vi "Set Lo Press.vi"(5 "Data.Direction":T1, 6 "leak":bool, 7 "init":bool, 8 "error in (no error)":errorcluster, 11 "Stand in":refnum<class "Stand.lvclass">) -> (0 "error out":errorcluster, 2 "Done":bool)   [LabVIEW 2019, in "Stand.lvclass"]
uses:
  Stand.lvclass
  C:/Users/ANENKOV_V1/Desktop/src/Device_class/Device.lvclass
  TypeDef/Direction.ctl
  Valve DIR.ctl
  Device_class/Device.lvclass/Device.ctl
  1305f1be-f95d-4b4d-845f-89e56356c3b4.vi
  Device_class/GetFPGA.vi
  DoValve.vi
  DoValve.vi/e7d2c9dc-ba67-4685-b926-bcce34aa2778.vi
  DoValve.vi/628819af-fd07-4303-9780-3ddd467101db.vi
  Const All Valve.vi
  FPGA_API_class/FPGA API.lvclass
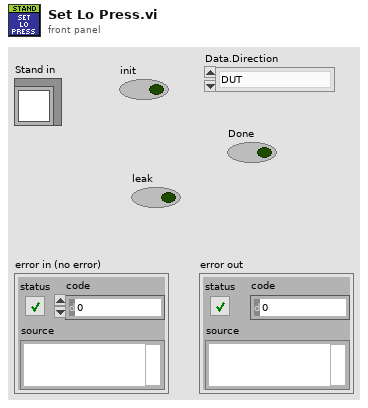
[diagram p1: front panel]
types:
  T1 = typedef "Direction.ctl" = enum8{"DUT", "Chamber"}
  T2 = typedef "Valve DIR.ctl" = enum16{"Air Valves: Open (DUT Filling)", "Air Valves: Open (Chamber Filling)", "Air Valves: Open (Pump Pressure DUT)", "Air Valves: Open (Pump Pressure Chamber)", "Air Valves: Open (Haskel Pressure DUT)", "Air Valves: Open (Haskel Pressure Chamber)", "Air Valves: Open (Slow Release DUT)", "Air Valves: Open (Slow Release Chamber)", "Air Valves: Open (Fast Release DUT)", "Air Valves: Open (Fast Release Chamber)", "Air Valves: Open (Emergency Release DUT and Chamber)", "Air Valves: Leak Hi (Chamber)", "Air Valves: Leak Hi (DUT)", "Air Valves: Backpressure (Chamber)", "Air Valves: Backpressure (DUT)", "Air Valves: Fully Closed", "Air Valves: Open 33.7"}
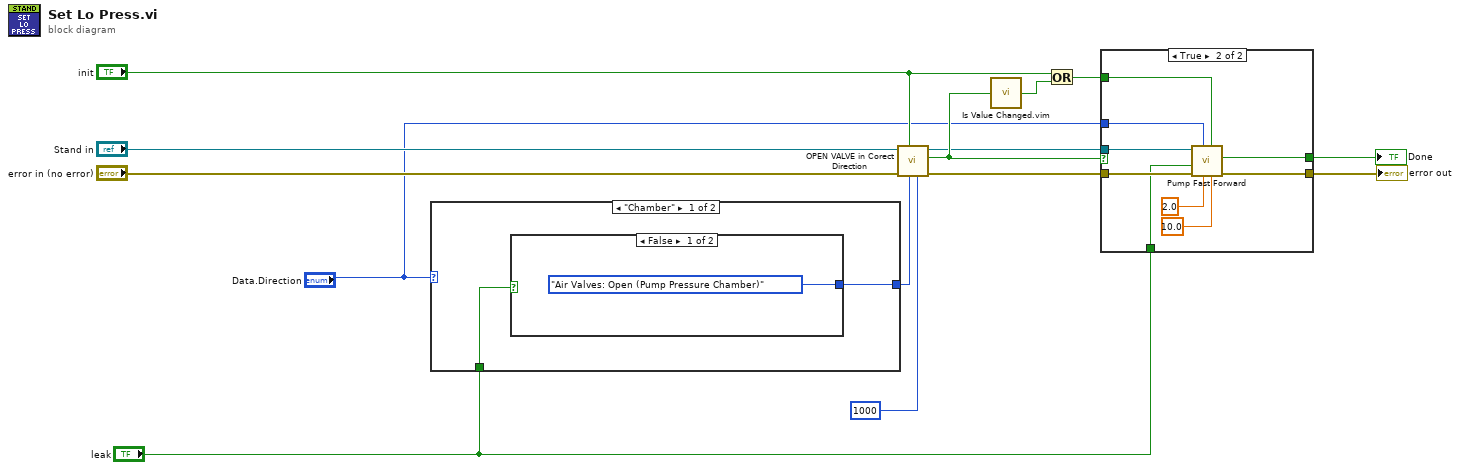
[diagram p0: block diagram]
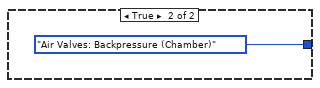
[diagram p3: hidden frame]
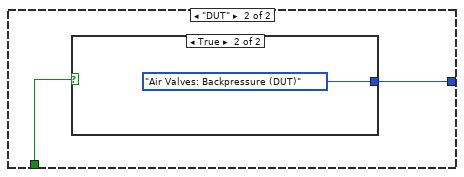
[diagram p4: hidden frame]
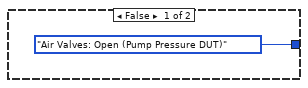
[diagram p5: hidden frame]
diagram:
  n1 = case shown="\"Chamber\"" "Data.Direction" {
    tunnel: [w16 w20] -> w4
    tunnel: "leak" -> [w15 w19]
    frame "Chamber" {
      n2 = case shown="False" w15 {
        tunnel: [Valve_DIR."Air Valves: Open (Pump Pressure Chamber)" ("Valve DIR") Valve_DIR."Air Valves: Backpressure (Chamber)" ("Valve DIR")] -> w16
        frame False {
        }
        frame True {
        }
      }
    }
    frame "DUT" {
      n3 = case shown="True" w19 {
        tunnel: [Valve_DIR."Air Valves: Open (Pump Pressure DUT)" ("Valve DIR") Valve_DIR."Air Valves: Backpressure (DUT)" ("Valve DIR")] -> w20
        frame False {
        }
        frame True {
        }
      }
    }
  }
  n4 = call "OPEN VALVE in Corect Direction.vi"("time after close"=u32 1000, "Valve DIR"=w4, "changed or first call?"="init", "error in (no error)"="error in (no error)", "Stand in"="Stand in") -> ("error out"=w7:errorcluster, "Done"=w11:bool, "Stand out"=w6:refnum<class "Stand.lvclass">)  [unwired: 4 in]
  n5 = call "Is Value Changed.vim"("value"=w11) -> ("changed or first call?"=w12:bool)
  n6 = Or(x="init", y=w12) -> (x .or. y?=w13:bool)
  n7 = case shown="True" w11 {
    tunnel: w6 -> [_ w32]
    tunnel: w7 -> [w23 w31]
    tunnel: [w23 w30] -> w8
    tunnel: w13 -> [_ w29]
    tunnel: [_ w28] -> w14
    tunnel: "Data.Direction" -> [_ w25]
    tunnel: "leak" -> [_ w24]
    frame False {
    }
    frame True {
      n8 = call "Pump Fast Forward.vi"("Time Target (s)"=10.0, "Init"=w29, "percent"=2.0, "Direction"=w25, "error in (no error)"=w31, "Leak"=w24, "Stand in"=w32) -> ("error out"=w30:errorcluster, "Done"=w28:bool)  [unwired: 3 in]
    }
  }
  "Done" <- w14
  "error out" <- w8
